vi "Update Void Command.vi"(8 "error in":errorcluster, 10 "Void":bool, 11 "CoreOOB_Tx in":refnum<class "CIFCoreOOB_Tx.lvclass">) -> (0 "error out":errorcluster, 3 "CoreOOB_Tx out":refnum<class "CIFCoreOOB_Tx.lvclass">)   [LabVIEW 2021, in "CIFCoreOOB_Tx.lvclass"]
uses:
  CIFCoreOOB_Tx.lvclass
  C:/Program Files/National Instruments/LabVIEW 2021/vi.lib/CIF Foundation/CIF Out of Band Commands/CIFOutOfBand.lvclass
  <vilib>/CIF Foundation/CIF Out of Band Commands/CIFOutOfBand.lvclass/CIFOutOfBand.ctl
  <vilib>/CIF Foundation/CIF Out of Band Commands/Typedef/OOB Container.ctl
  Typedef/Template Payload.ctl
  Typedef/OOB Core Commands.ctl
  CIFCoreOOB_Tx.lvclass/CIFCoreOOB_Tx.ctl
  <vilib>/CIF Foundation/CIF Out of Band Commands/CIFOutOfBand.lvclass
  D:/dev/CIF-LVCore/src/CIFCore/OOB/OOB_Tx/CIFCoreOOB_Tx.lvclass
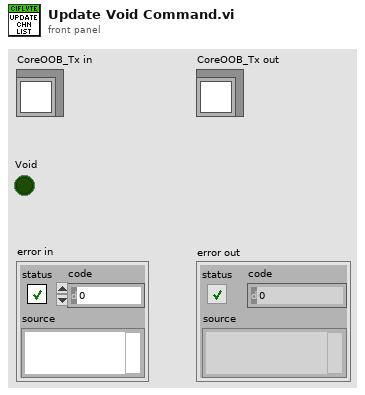
[diagram p1: front panel]
types:
  T1 = typedef "CIFOutOfBand.lvclass/OOB Container.ctl" = cluster{"Commands (bitwise)":u64, "Payload":variant}
  T2 = typedef "CIFCoreOOB_Tx.lvclass/Template Payload.ctl" = cluster{"void":bool}
  T3 = typedef "CIFCoreOOB_Tx.lvclass/OOB Core Commands.ctl" = enum8{"void"}
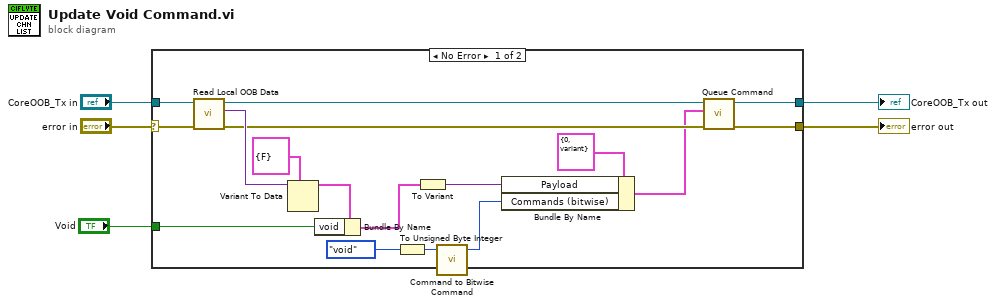
[diagram p0: block diagram]
diagram:
  n1 = case shown="No Error" "error in" {
    selector: "error in" -> [w20 w24]
    tunnel: [w21 w24] -> w4
    tunnel: "CoreOOB_Tx in" -> [w19 w23]
    tunnel: [w22 w23] -> w2
    tunnel: "Void" -> [w12 _]
    frame No Error {
      n2 = call <vilib>:"Read Local OOB Data.vi"("error in"=w20, "OOB in"=w19) -> ("error out"=w9:errorcluster, "Local OOB Data"=w14:variant, "OOB out"=w8:refnum<class "CIFCoreOOB_Tx.lvclass">)  [unwired: 7 in]
      n3 = Variant To Data(type=T2 {"void"=FALSE} ("Template Payload"), Variant=w14) -> (data=w16:T2)  [unwired: 1 in, 1 out]
      n4 = Bundle By Name(cluster=w16, "void"=w12) -> (w15:T2)
      n5 = To Unsigned Byte Integer(number=OOB_Core_Commands."void" ("OOB Main Commands")) -> (unsigned 8bit integer=w18:u8)
      n6 = To Variant(anything=w15) -> (Variant=w10:variant)
      n7 = call <vilib>:"Command to Bitwise Command.vi"("Command"=w18) -> ("bit command"=w7:u64)  [unwired: 3 in]
      n8 = Bundle By Name(cluster=T1 {"Commands (bitwise)"=0, "Payload"=variant} ("OOB Data"), "Payload"=w10, "Commands (bitwise)"=w7) -> (w6:T1)
      n9 = call <vilib>:"Queue Command.vi"("error in"=w9, "OOB Data"=w6, "OOB in"=w8) -> ("error out"=w21:errorcluster, "OOB out"=w22:refnum<class "CIFCoreOOB_Tx.lvclass">)  [unwired: 7 in]
    }
    frame Error {
    }
  }
  "error out" <- w4
  "CoreOOB_Tx out" <- w2
